vi "Auto - Drive a Distance.vi"(9 "Auton Cluster In":T2, 11 "Auton State In":i32) -> (1 "Auton Cluster Out":T2, 3 "Auton State Out":i32, 4 "Strafe Y (ROBOT)":dbl, 6 "Strafe X (ROBOT)":dbl)   [LabVIEW 2020]
uses:
  TypeDefs/Auton Cluster Typedef.ctl
  Team Code/Robot Global Data.vi
  <vilib>/addons/control/pid/pid.llb/PID (DBL).vi
  <vilib>/addons/control/pid/NI_PID_pid.lvlib
panel:
  in  "YPID gains":T1={"proportional gain (Kc)"=0.65, "integral time (Ti, min)"=0.0, "derivative time (Td, min)"=0.0} {"derivative time (Td, min)" format="%.3f"; "integral time (Ti, min)" format="%.3f"; "proportional gain (Kc)" format="%.3f"}
  in  "XPID gains":T1={"proportional gain (Kc)"=0.65, "integral time (Ti, min)"=0.0, "derivative time (Td, min)"=0.0} {"derivative time (Td, min)" format="%.3f"; "integral time (Ti, min)" format="%.3f"; "proportional gain (Kc)" format="%.3f"}
  in  "Minimum":dbl=0.2
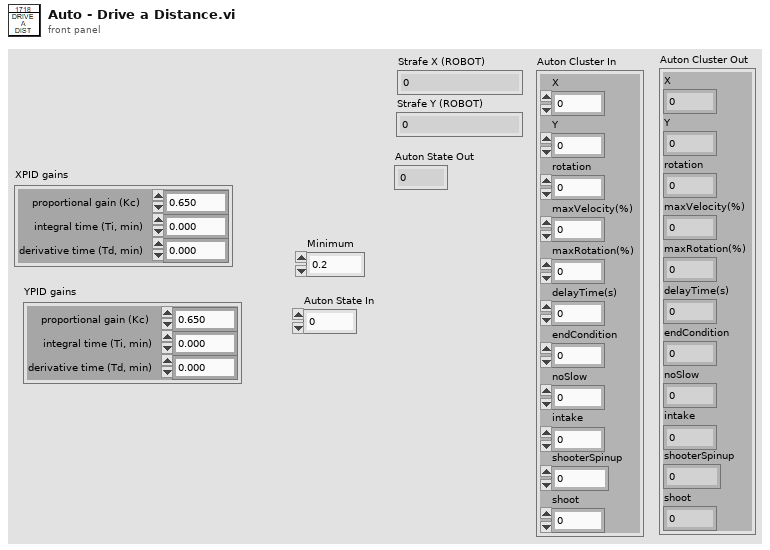
[diagram p1: front panel]
types:
  T1 = cluster{"proportional gain (Kc)":dbl, "integral time (Ti, min)":dbl, "derivative time (Td, min)":dbl}
  T2 = typedef "Auton Cluster Typedef.ctl" = cluster{"rotation":dbl, "maxVelocity(%)":dbl, "delayTime(s)":dbl, "endCondition":dbl, "noSlow":dbl, "intake":dbl, "shooterSpinup":dbl, "shoot":dbl, "X":dbl, "Y":dbl, "maxRotation(%)":dbl}
  T3 = typedef "Trajectory_Library.lvlib/SWERVE_DRIVE_ODOMETRY.ctl" = cluster{"POSE":T4, "GyroOffset":T6, "PreviousAngle":T6, "PrevTime":dbl}
  T4 = typedef "Trajectory_Library.lvlib/POSE2D.ctl" = cluster{"TRANSLATION":T5, "ROTATION":T6}
  T5 = typedef "Trajectory_Library.lvlib/TRANSLATION2D.ctl" = cluster{"X":dbl, "Y":dbl}
  T6 = typedef "Trajectory_Library.lvlib/ROTATION2D.ctl" = cluster{"VALUE":dbl, "COS":dbl, "SIN":dbl}
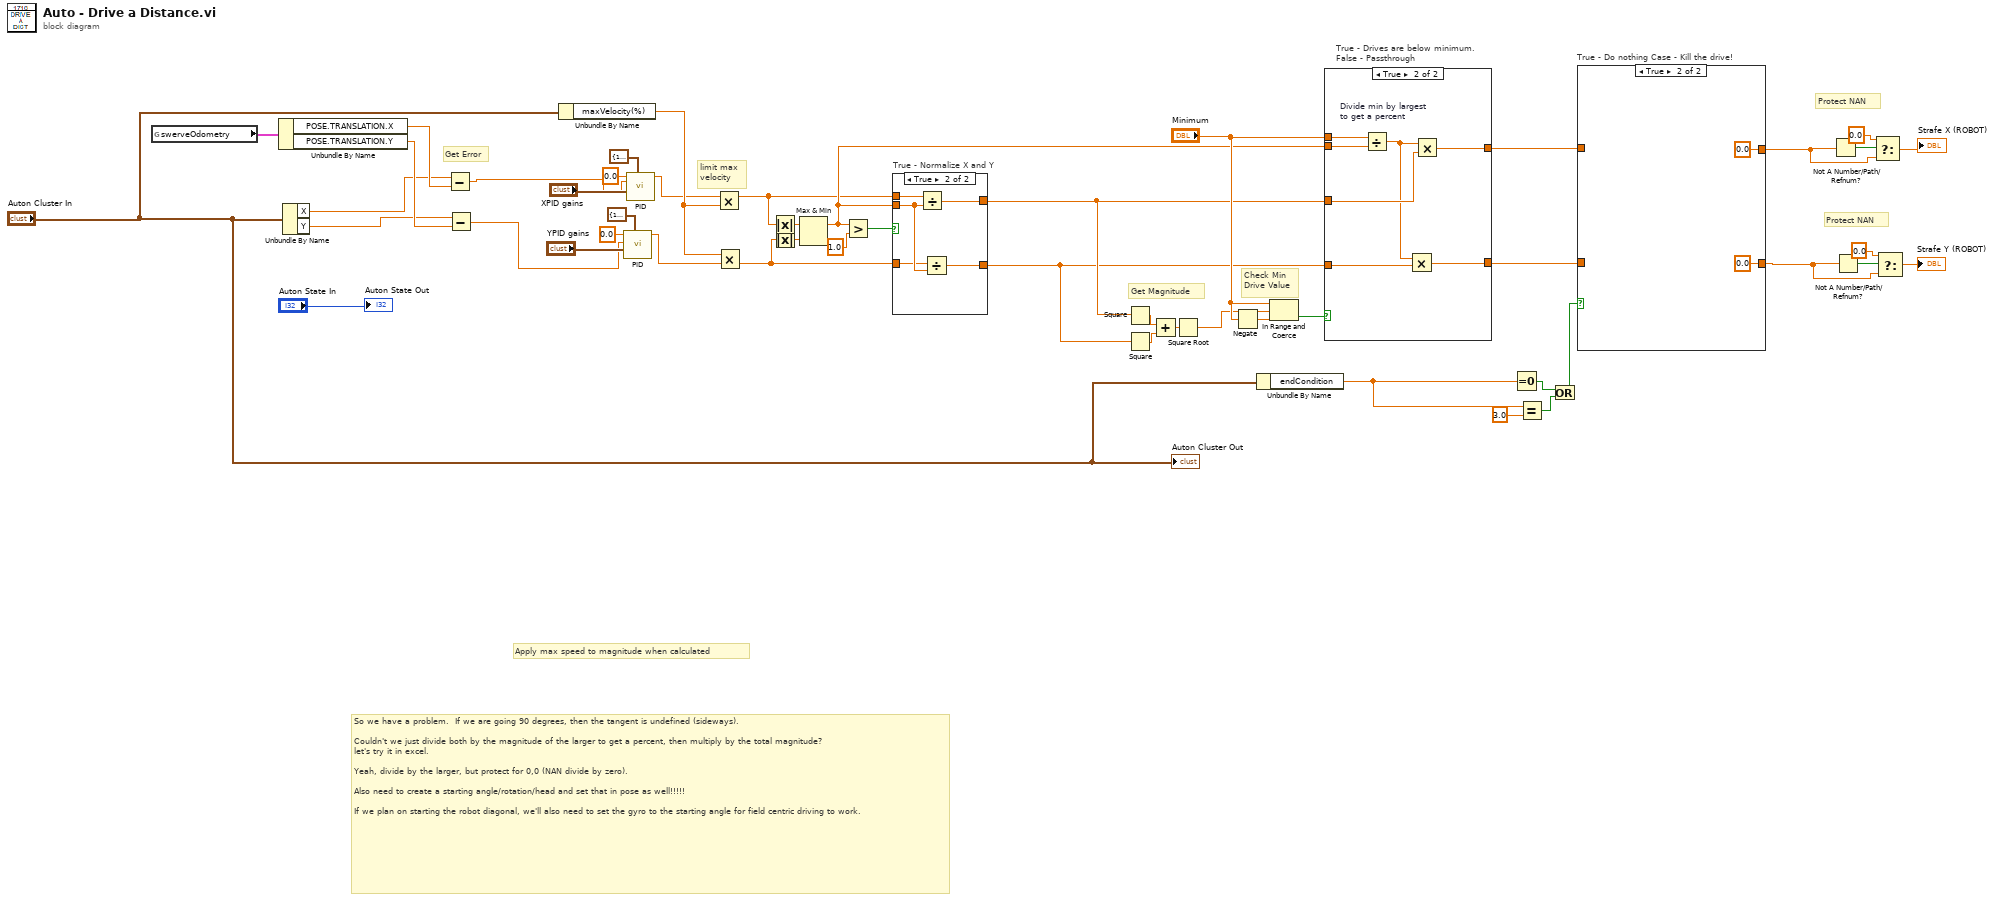
[diagram p0: block diagram]
diagram:
  # "limit max\nvelocity"
  # "Check Min\nDrive Value"
  # "Get Magnitude"
  # "Protect NAN"
  # "Protect NAN"
  # "Get Error"
  # "So we have a problem.  If we are going 90 degrees, then the tangent is undefined (sideways).\n\nCouldn't we just divide both by the magnitude of the larger to get a percent, then multiply by the total magnitude?\nlet's try it in excel.\n\nYeah, divide by the larger, but protect for 0,0 (NAN divide by zero).\n\nAlso need to create a starting angle/rotation/head and set that in pose as well!!!!!\n\nIf we plan on starting the robot diagonal, we'll also need to set the gyro to the starting angle for field centric driving to work."
  # "Apply max speed to magnitude when calculated"
  n1 = global read "Robot Global Data.vi" "swerveOdometry"() -> (w47:T3)
  n2 = Unbundle By Name(w47) -> ("POSE.TRANSLATION.X"=w49:dbl, "POSE.TRANSLATION.Y"=w48:dbl)
  n3 = Unbundle By Name("Auton Cluster In") -> ("X"=w45:dbl, "Y"=w46:dbl)
  n4 = Subtract(x=w45, y=w49) -> (x-y=w6:dbl)
  n5 = Subtract(x=w46, y=w48) -> (x-y=w2:dbl)
  n6 = Unbundle By Name("Auton Cluster In") -> ("maxVelocity(%)"=w21:dbl)
  n7 = call-poly <vilib>:"PID.vi"("output range"=cluster{"output high":dbl, "output low":dbl} {"output high"=1.0, "output low"=-1.0}, "PID gains"="YPID gains", "process variable"=w2, "setpoint"=0.0) -> ("output"=w1:dbl)  [unwired: 6 in, 1 out]
  n8 = call-poly <vilib>:"PID.vi"("output range"=cluster{"output high":dbl, "output low":dbl} {"output high"=1.0, "output low"=-1.0}, "PID gains"="XPID gains", "process variable"=w6, "setpoint"=0.0) -> ("output"=w7:dbl)  [unwired: 6 in, 1 out]
  n9 = Multiply(x=w7, y=w21) -> (x*y=w23:dbl)
  n10 = Multiply(x=w21, y=w1) -> (x*y=w22:dbl)
  n11 = Absolute Value(x=w23) -> (abs(x)=w38:dbl)
  n12 = Absolute Value(x=w22) -> (abs(x)=w37:dbl)
  n13 = Max & Min(x=w38, y=w37) -> (max(x,y)=w26:dbl)  [unwired: 1 out]
  n14 = Greater?(x=w26, y=1.0) -> (0:w39:bool)
  n15 = case "True - Normalize X and Y" shown="True" w39 {
    tunnel: w22 -> [w50 w54]
    tunnel: w23 -> [w51 w56]
    tunnel: w26 -> [_ w55]
    tunnel: [w51 w53] -> w28
    tunnel: [w50 w52] -> w27
    frame False {
    }
    frame True {
      n16 = Divide(x=w56, y=w55) -> (x/y=w53:dbl)
      n17 = Divide(x=w54, y=w55) -> (x/y=w52:dbl)
    }
  }
  n18 = Square(x=w28) -> (x^2=w35:dbl)
  n19 = Square(x=w27) -> (x^2=w36:dbl)
  n20 = Add(x=w35, y=w36) -> (x+y=w34:dbl)
  n21 = Square Root(x=w34) -> (sqrt(x)=w33:dbl)
  n22 = Negate(x="Minimum") -> (-x=w43:dbl)
  n23 = Unbundle By Name("Auton Cluster In") -> ("endCondition"=w12:dbl)
  n24 = In Range and Coerce(upper limit="Minimum", x=w33, lower limit=w43) -> (In Range?=w41:bool)  [unwired: 1 out]
  n25 = case "True - Drives are below minimum.\nFalse - Passthrough" shown="True" w41 {
    tunnel: [w57 w65] -> w20
    tunnel: [w58 w64] -> w19
    tunnel: "Minimum" -> [_ w63]
    tunnel: w28 -> [w57 w61]
    tunnel: w27 -> [w58 w60]
    tunnel: w26 -> [_ w62]
    frame False {
    }
    frame True {
      n26 = Divide "Divide min by largest\nto get a percent"(x=w63, y=w62) -> (x/y=w59:dbl)
      n27 = Multiply(x=w59, y=w60) -> (x*y=w64:dbl)
      n28 = Multiply(x=w59, y=w61) -> (x*y=w65:dbl)
    }
  }
  n29 = Equal To 0?(x=w12) -> (x = 0?=w15:bool)
  n30 = Equal?(x=w12, y=3.0) -> (x = y?=w13:bool)
  n31 = Or(x=w15, y=w13) -> (x .or. y?=w14:bool)
  n32 = case "True - Do nothing Case - Kill the drive!" shown="True" w14 {
    tunnel: w20 -> [w67 _]
    tunnel: w19 -> [w66 _]
    tunnel: [w67 0.0] -> w18
    tunnel: [w66 0.0] -> w17
    frame False {
    }
    frame True {
    }
  }
  n33 = Not A Number/Path/Refnum?(number/path/refnum=w18) -> (NaN/Path/Refnum?=w32:bool)
  n34 = Not A Number/Path/Refnum?(number/path/refnum=w17) -> (NaN/Path/Refnum?=w29:bool)
  n35 = Select(t=0.0, s=w32, f=w18) -> (s? t:f=→"Strafe X (ROBOT)":dbl)
  n36 = Select(t=0.0, s=w29, f=w17) -> (s? t:f=→"Strafe Y (ROBOT)":dbl)
  "Auton Cluster Out" <- "Auton Cluster In"
  "Auton State Out" <- "Auton State In"
